vi "jsoncheck2016.vi"() -> ()   [LabVIEW 2016]
panel:
  out "value 2":T1
  in  "Boolean":bool=TRUE
  out "value":T2
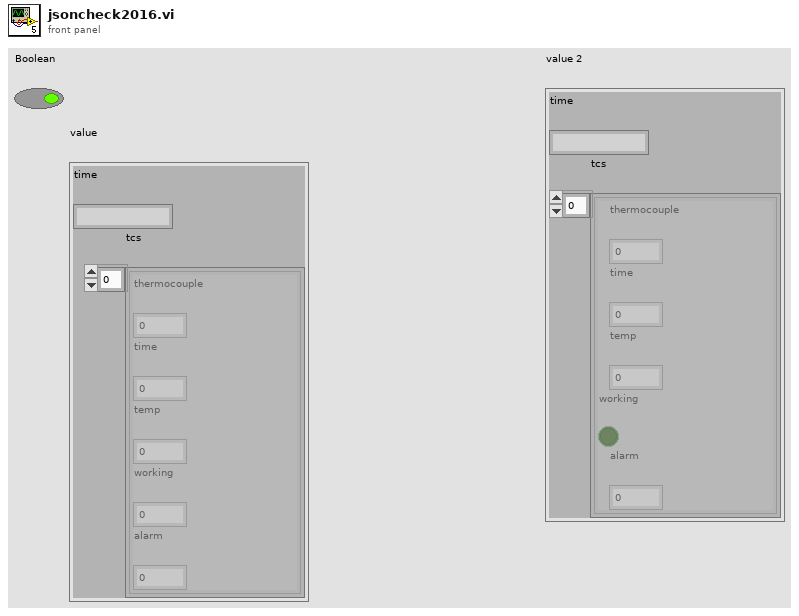
[diagram p1: front panel]
types:
  T1 = cluster{"time":string, "tcs":cluster{"thermocouple":i32, "time":i32, "temp":i32, "working":bool, "alarm":i32}[]}
  T2 = cluster{"time":string, "tcs":cluster{"thermocouple":i32, "time":i32, "temp":i32, "working":i32, "alarm":i32}[]}
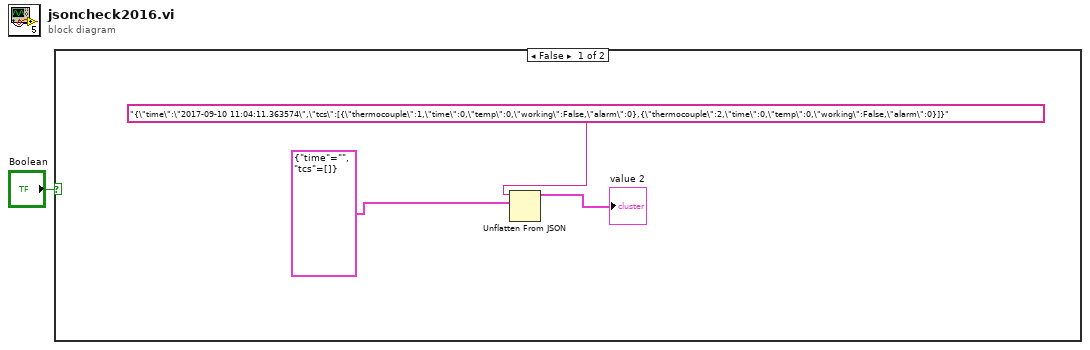
[diagram p0: block diagram]
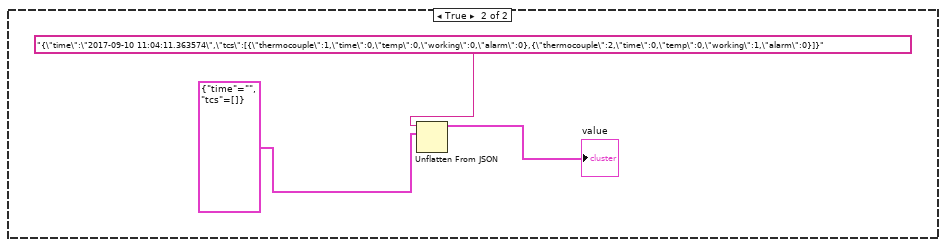
[diagram p2: hidden frame]
diagram:
  n1 = case shown="False" "Boolean" {
    frame False {
      n2 = Unflatten From JSON(JSON string="{\"time\":\"2017-09-10 11:04:11.363574\",\"tcs\":[{\"thermocouple\":1,\"time\":0,\"temp\":0,\"working\":False,\"alarm\":0},{\"thermocouple\":2,\"time\":0,\"temp\":0,\"working\":False,\"alarm\":0}]}", type and defaults=T1 {"time"="", "tcs"=[]} ("Cluster")) -> (value=→"value 2":T1)  [unwired: 5 in, 1 out]
    }
    frame True {
      n3 = Unflatten From JSON(JSON string="{\"time\":\"2017-09-10 11:04:11.363574\",\"tcs\":[{\"thermocouple\":1,\"time\":0,\"temp\":0,\"working\":0,\"alarm\":0},{\"thermocouple\":2,\"time\":0,\"temp\":0,\"working\":1,\"alarm\":0}]}", type and defaults=T2 {"time"="", "tcs"=[]} ("Cluster")) -> (value=→"value":T2)  [unwired: 5 in, 1 out]
    }
  }
